vi "Plot axes format string.vi"(7 "TimeZone":T1, 8 "error in (no error)":errorcluster, 10 "Scale reference":refnum<vi>, 11 "Meta LUT":refnum<data-value>) -> (0 "error out":errorcluster, 2 "Scale reference":refnum<vi>)   [LabVIEW 2021, in "RocketPlot.lvlib"]
uses:
  RocketPlot.lvlib
  TypeDefs/TimeZone.ctl
  Plot scale refnum to LUT name.vi
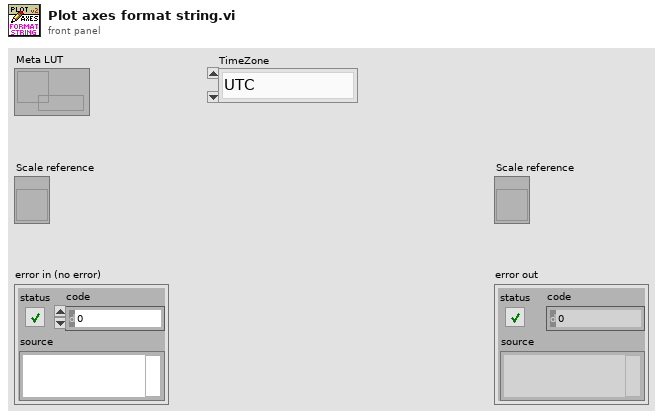
[diagram p1: front panel]
types:
  T1 = typedef "RocketPlot.lvlib/TimeZone.ctl" = enum16{"UTC", "Local"}
  T2 = typedef "RocketPlot.lvlib/Plot scale meta JSON.ctl" = cluster{"Type":T3, "Grid Colors:Major Color":u32, "Grid Colors:Minor Color":u32, "Style":u8, "Tick Colors:Tick Color":u32, "Tick Colors:Minor Tick Color":u32, "Format String":string, "State":T4, "AxisFocus":refnum<vi>}
  T3 = typedef "RocketPlot.lvlib/Plot axis.ctl" = enum16{"x axis", "left axis", "right axis"}
  T4 = typedef "RocketPlot.lvlib/Plot scale meta state.ctl" = cluster{"Visible":bool, "Focus":bool, "Multi-Y":bool}
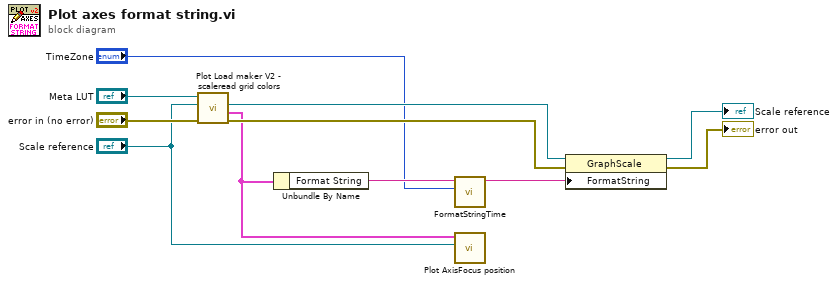
[diagram p0: block diagram]
diagram:
  n1 = call "Plot Load maker V2 - scaleread grid colors.vi"("error in (no error)"="error in (no error)", "Scale reference"="Scale reference", "Meta LUT"="Meta LUT") -> ("error out"=w9:errorcluster, "Scale LUT meta"=w2:T2, "Scale reference"=w10:refnum<vi>)  [unwired: 5 in, 1 out]
  n2 = Unbundle By Name(w2) -> ("Format String"=w5:string)
  n3 = call "FormatStringTime.vi"("TimeZone"="TimeZone", "Format String"=w5) -> ("Format String"=w4:string)  [unwired: 9 in]
  n4 = call "Plot AxisFocus position.vi"("Scale reference"="Scale reference", "Scale LUT meta"=w2) -> ()  [unwired: 9 in, 1 out]
  n5 = property class="GraphScale"(reference=w10, error in=w9, "FormatString"=w4) -> (reference out=→"Scale reference":refnum<vi>, error out=→"error out":errorcluster)
